vi "Chronos TDMS Viewer Read End Time.vi"(8 "error in (no error)":errorcluster, 10 "group name":string, 11 "tdms file":refnum<k34>) -> (0 "error out":errorcluster, 1 "end time":timestamp, 2 "group name dup":string, 3 "tdms file dup":refnum<k34>)   [LabVIEW 2021]
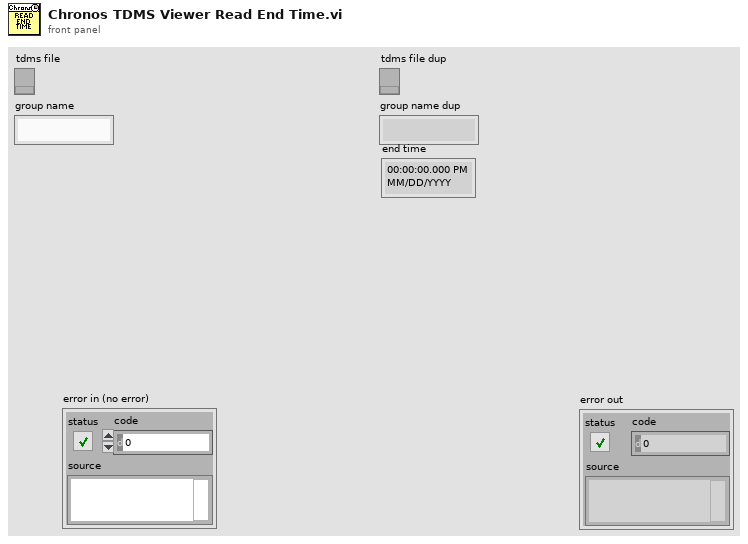
[diagram p1: front panel]
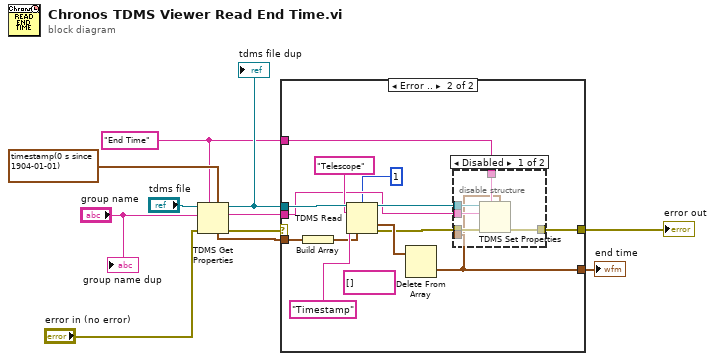
[diagram p0: block diagram]
diagram:
  w4 = "End Time" ("group name")
  n1 = TDMS Get Properties(5:timestamp(0 s since 1904-01-01), 7:w4, 8:"error in (no error)", 10:"group name", 11:"tdms file") -> (0:w1:errorcluster, 2:w7:string, 3:w8:refnum<k34>, 4:w3:timestamp)  [unwired: 1 in, 2 out]
  "tdms file dup" <- w8
  n2 = case shown="Error .." w1 {
    selector: w1 -> [w12 _]
    tunnel: w8 -> [_ w26]
    tunnel: w7 -> [_ w21]
    tunnel: w3 -> [w13 w16]
    tunnel: w4 -> [_ w20]
    tunnel: [w12 w18] -> w6
    tunnel: [w13 w14] -> w2
    frame No Error {
    }
    frame Error {
      (unwired) string[] []
      n3 = Build Array(w16) -> (w15:timestamp[])
      n4 = TDMS Read(0:w26, 2:i64 1 ("count (-1: all)"), 5:"Telescope" ("group name"), 7:"Timestamp" ("group name"), 12:w15) -> (4:w23:refnum<k34>, 10:w24:timestamp[], 15:w19:errorcluster)  [unwired: 3 in, 3 out]
      n5 = Delete From Array(array=w24) -> (deleted portion=w14:timestamp)  [unwired: 2 in, 1 out]
      n6 = disable-structure shown="Disabled" {
        disable-tunnel: w23 -> [w32 _]
        disable-tunnel: w21 -> [w31 _]
        disable-tunnel: w20 -> [w30 _]
        disable-tunnel: w19 -> [w29 w33]
        disable-tunnel: [w28 w33] -> w18
        disable-tunnel: w14 -> [w27 _]
        frame Disabled {
          n7 = TDMS Set Properties(5:w27, 7:w30, 8:w29, 10:w31, 11:w32) -> (0:w28:errorcluster)  [unwired: 1 in, 3 out]
        }
        frame Enabled {
        }
      }
    }
  }
  "error out" <- w6
  "end time" <- w2
  "group name dup" <- "group name"
